vi "MyQueue.vi"(7 "Mode":T1(ring), 8 "error in (no error)":errorcluster, 10 "Queue In":string) -> (0 "error out":errorcluster, 2 "Queue Out":string)   [LabVIEW 2011]
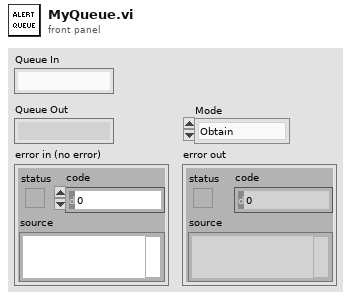
[diagram p1: front panel]
types:
  T1 = enum16{"Obtain", "Enqueue", "Dequeue", "Release"}
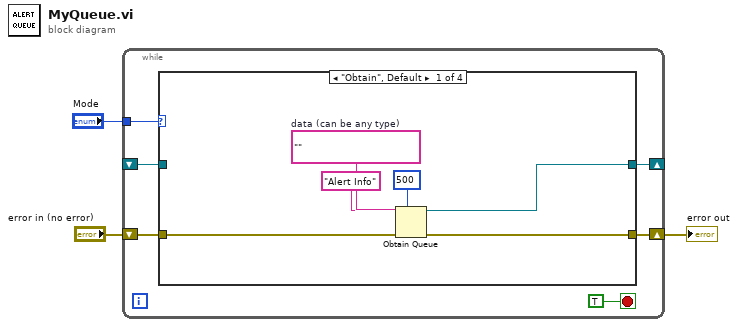
[diagram p0: block diagram]
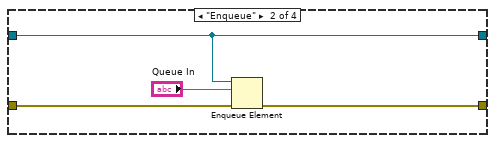
[diagram p2: hidden frame]
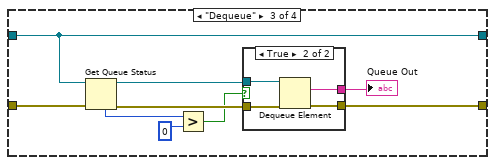
[diagram p3: hidden frame]
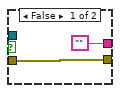
[diagram p4: hidden frame]
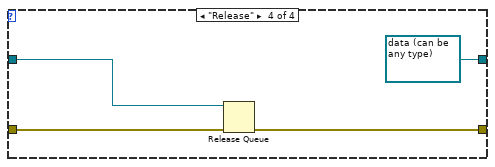
[diagram p5: hidden frame]
diagram:
  n1 = while {
    tunnel: "Mode" -> [w9]
    shift-right: [w7] -> w1
    shift-left: "error in (no error)" -> [w8]
    shift-right: [w6] -> _
    shift-left: _ -> [w5]
    stop <- TRUE stop-if-true
    n2 = case shown="\"Obtain\", Default" w9 {
      tunnel: w8 -> [w15 w19 w26 w38]
      tunnel: [w14 w18 w28 w37] -> w7
      tunnel: [w11 w16 w24 refnum<queue> refnum ("queue out")] -> w6
      tunnel: w5 -> [_ w16 w24 w36]
      frame "Obtain", Default {
        w13 = ""  # data (can be any type)
        n3 = Obtain Queue(max queue size (-1, unlimited)=500, name (unnamed)="Alert Info", element data type=w13, error in (no error)=w15) -> (queue out=w11:refnum<queue>, error out=w14:errorcluster)  [unwired: 1 in, 1 out]
      }
      frame "Enqueue" {
        n4 = Enqueue Element(queue=w16, element="Queue In", error in (no error)=w19) -> (error out=w18:errorcluster)  [unwired: 1 in, 2 out]
      }
      frame "Dequeue" {
        n5 = Get Queue Status(queue=w24, error in (no error)=w26) -> (queue out=w23:refnum<queue>, error out=w25:errorcluster, # elements in queue=w21:i32)  [unwired: 1 in, 5 out]
        n6 = Greater?(x=w21, y=0) -> (0:w20:bool)
        n7 = case shown="True" w20 {
          tunnel: [w29 w34] -> w28
          tunnel: ["" w33] -> w27
          tunnel: w25 -> [w29 w32]
          tunnel: w23 -> [_ w31]
          frame False {
          }
          frame True {
            n8 = Dequeue Element(queue=w31, error in (no error)=w32) -> (element=w33:string, error out=w34:errorcluster)  [unwired: 1 in, 2 out]
          }
        }
        "Queue Out" <- w27
      }
      frame "Release" {
        n9 = Release Queue(queue=w36, error in (no error)=w38) -> (error out=w37:errorcluster)  [unwired: 1 in, 2 out]
      }
    }
  }
  "error out" <- w1
